vi "Traffic Light.vi"() -> ()   [LabVIEW 2022 SP3]
uses:
  Traffic Light.ctl
panel:
  in  "stop":bool
  out "Green":bool
  out "Red":bool
  out "Yellow":bool
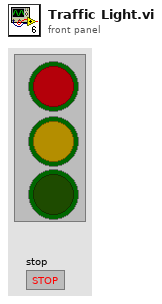
[diagram p1: front panel]
types:
  T1 = typedef "Traffic Light.ctl" = enum16{"Green", "Yellow", "Red", ""}
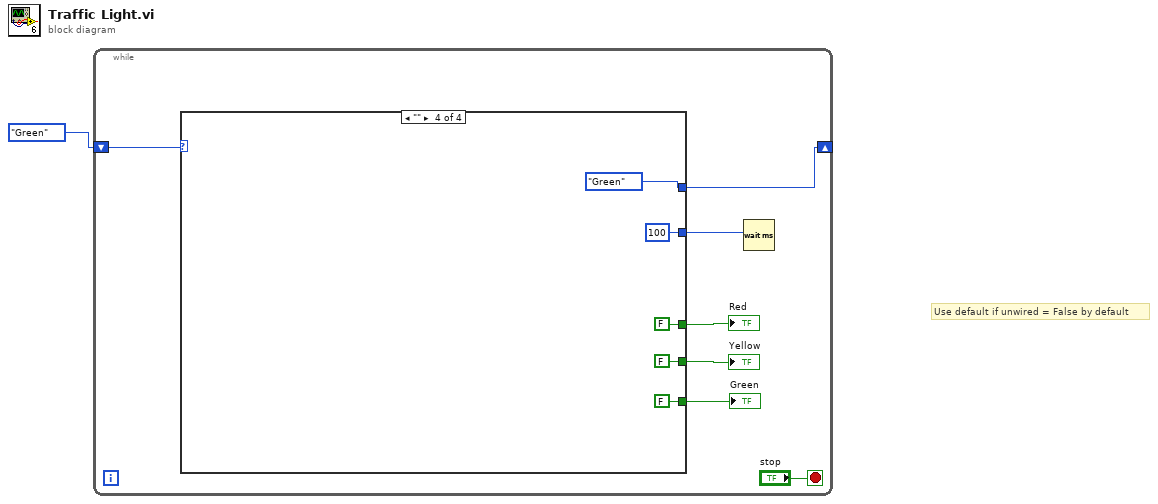
[diagram p0: block diagram]
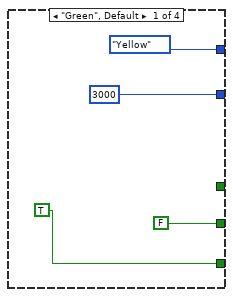
[diagram p2: hidden frame]
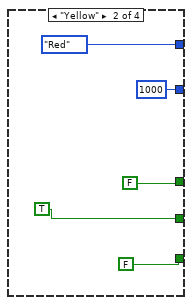
[diagram p3: hidden frame]
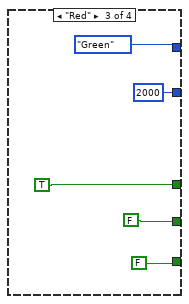
[diagram p4: hidden frame]
diagram:
  # "Use default if unwired = False by default"
  n1 = while {
    shift-right: [w3] -> _
    shift-left: Traffic_Light."Green" -> [w7]
    stop <- "stop" stop-if-true
    n2 = case shown="\"\"" w7 {
      tunnel: [_ FALSE TRUE FALSE] -> w6
      tunnel: [FALSE TRUE FALSE FALSE] -> w5
      tunnel: [TRUE FALSE FALSE FALSE] -> w4
      tunnel: [Traffic_Light."Yellow" Traffic_Light."Red" Traffic_Light."Green" Traffic_Light."Green"] -> w3
      tunnel: [u32 3000 ("milliseconds to wait") u32 1000 ("milliseconds to wait") u32 2000 ("milliseconds to wait") u32 100 ("milliseconds to wait")] -> w2
      frame "Green", Default {
      }
      frame "Yellow" {
      }
      frame "Red" {
      }
      frame "" {
      }
    }
    "Green" <- w4
    "Yellow" <- w5
    "Red" <- w6
    n3 = Wait (ms)(milliseconds to wait=w2) -> ()  [unwired: 1 out]
  }
